vi "ECG_GetFilterProgress.vi"(8 "error in (no error)":errorcluster caption="错误输入（无错误）", 10 "target length":i32 caption="目标长度", 11 "current length":i32 caption="当前长度") -> (0 "error out":errorcluster caption="错误输出", 2 "done":bool caption="完成", 3 "progress":u8 caption="进度")   [LabVIEW 2022 SP3]
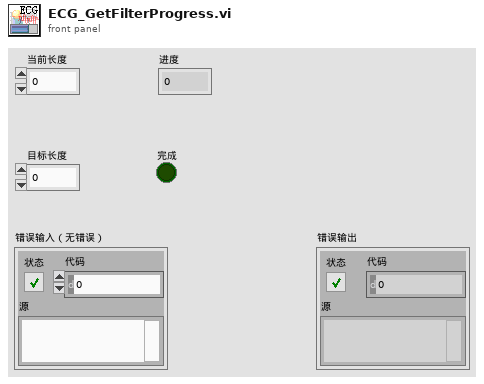
[diagram p1: front panel]
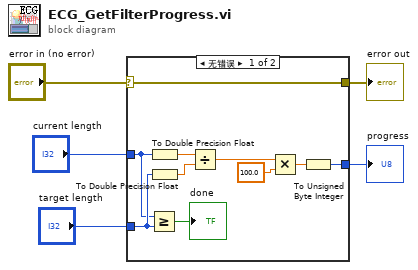
[diagram p0: block diagram]
diagram:
  n1 = case shown="无错误" "error in (no error)" {
    selector: "error in (no error)" -> [w6 w16]
    tunnel: "target length" -> [w15 _]
    tunnel: "current length" -> [w14 _]
    tunnel: [w13 _] -> w3
    tunnel: [w6 w16] -> w1
    frame No Error {
      n2 = Greater Or Equal?(x=w14, y=w15) -> (x >= y?=→"done":bool)
      n3 = To Double Precision Float(number=w14) -> (double precision float=w8:dbl)
      n4 = To Double Precision Float(number=w15) -> (double precision float=w9:dbl)
      n5 = Divide(x=w8, y=w9) -> (x/y=w11:dbl)
      n6 = Multiply(x=w11, y=100.0) -> (x*y=w10:dbl)
      n7 = To Unsigned Byte Integer(number=w10) -> (unsigned 8bit integer=w13:u8)
    }
    frame Error {
    }
  }
  "progress" <- w3
  "error out" <- w1
